vi "PixieReadRunTime.vi"(8 "error in (no error)":errorcluster, 9 "Module number":u16 max=17 step=1) -> (0 "error out":errorcluster, 1 "Run time [s]":dbl)   [LabVIEW 2013]
uses:
  XIA/Pixie4/Drivers/Pixie4DLL.dll
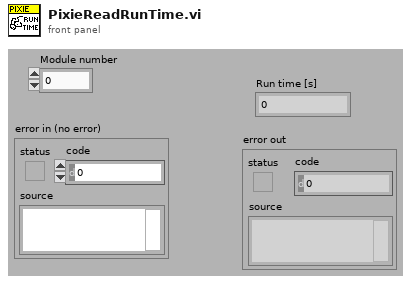
[diagram p1: front panel]
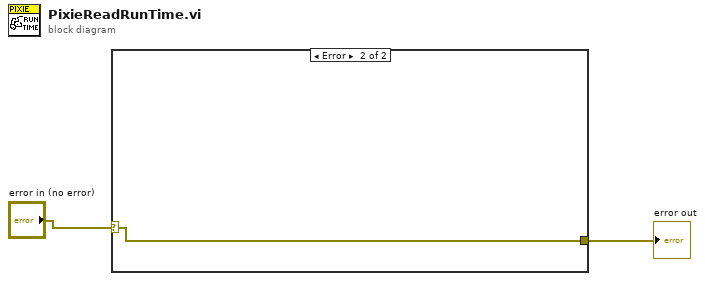
[diagram p0: block diagram]
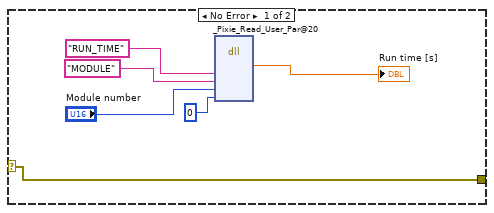
[diagram p2: hidden frame]
diagram:
  n1 = case shown="Error" "error in (no error)" {
    selector: "error in (no error)" -> [w3 w9]
    tunnel: [w3 w9] -> w1
    frame No Error {
      n2 = dll-call lib="C:/XIA/Pixie4/Drivers/Pixie4DLL.dll" fn="_Pixie_Read_User_Par@20"("User_Par_Name"="RUN_TIME", "User_Par_Type"="MODULE", "ModNum"="Module number", "ChanNum"=0) -> ("User_Par_Value"=→"Run time [s]":dbl)  [unwired: 4 in, 7 out]
    }
    frame Error {
    }
  }
  "error out" <- w1
